vi "Init.vi"(8 "error in (no error)":errorcluster, 11 "Profile Name":string) -> (0 "error out":errorcluster, 3 "CreateProfile out":refnum<class "CreateProfile.lvclass">)   [LabVIEW 2022 SP3, in "obs-websocket-lv.lvlib" / "CreateProfile.lvclass"]
uses:
  CreateProfile.lvclass
  CreateProfile.lvclass/CreateProfile.ctl
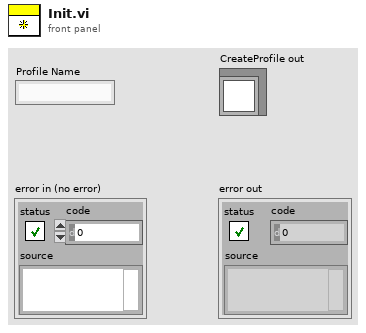
[diagram p1: front panel]
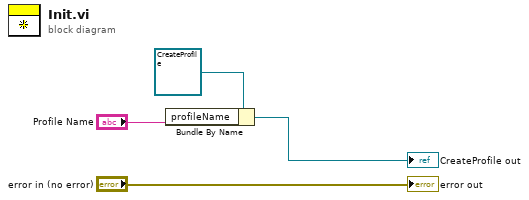
[diagram p0: block diagram]
diagram:
  n1 = Bundle By Name(cluster=refnum<class "CreateProfile.lvclass"> refnum ("CreateProfile in"), "profileName"="Profile Name") -> (→"CreateProfile out":refnum<class "CreateProfile.lvclass">)
  "error out" <- "error in (no error)"
